vi "boolean 3.vi"() -> ()   [LabVIEW 2025]
panel:
  out "Boolean 8":bool
  out "Boolean 7":bool
  out "Boolean 6":bool
  out "Boolean 5":bool
  out "Boolean 4":bool
  out "Boolean 3":bool
  in  "Boolean 2":bool
  in  "Boolean":bool
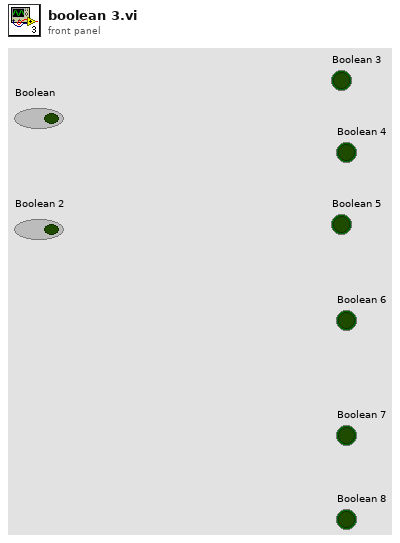
[diagram p1: front panel]
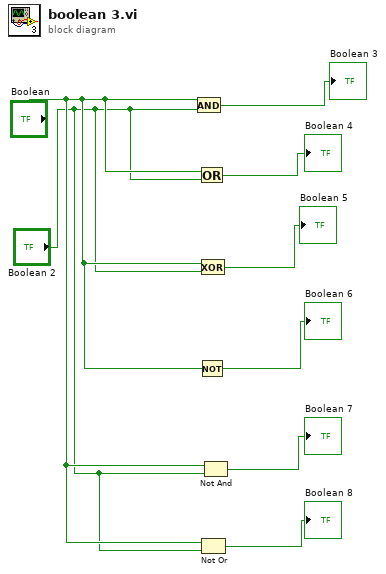
[diagram p0: block diagram]
diagram:
  n1 = And(x="Boolean", y="Boolean 2") -> (x .and. y?=→"Boolean 3":bool)
  n2 = Or(x="Boolean", y="Boolean 2") -> (x .or. y?=→"Boolean 4":bool)
  n3 = Not(x="Boolean") -> (.not. x?=→"Boolean 6":bool)
  n4 = Exclusive Or(1:"Boolean 2", 2:"Boolean") -> (0:→"Boolean 5":bool)
  n5 = Not Or(1:"Boolean 2", 2:"Boolean") -> (0:→"Boolean 8":bool)
  n6 = Not And(1:"Boolean 2", 2:"Boolean") -> (0:→"Boolean 7":bool)
